vi "Close Handle.vi"(8 "error in (no error)":errorcluster, 11 "HTTP Client Base in":refnum<class "HTTP Client Base.lvclass">) -> (0 "error out":errorcluster, 3 "HTTP Client Base out":refnum<class "HTTP Client Base.lvclass">)   [LabVIEW 2021, in "HTTP Client Base.lvclass"]
uses:
  HTTP Client Base.lvclass
  HTTP Client Base.lvclass/HTTP Client Base.ctl
  <vilib>/httpClient/ClientHandle.ctl
  <vilib>/httpClient/LabVIEWHTTPClient.lvlib
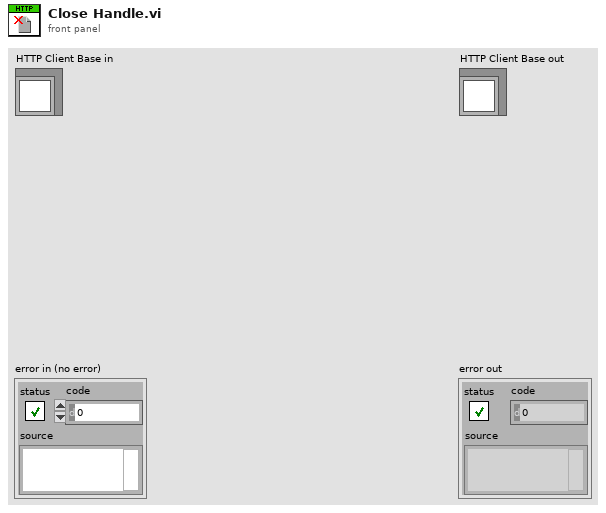
[diagram p1: front panel]
types:
  T1 = typedef "LabVIEWHTTPClient.lvlib/ClientHandle.ctl" = refnum<k1>
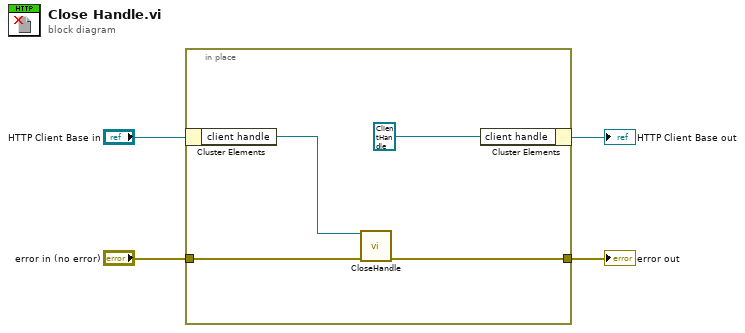
[diagram p0: block diagram]
diagram:
  n1 = in-place {
    in-place-border: "error in (no error)" -> [w8]
    in-place-border: [w7] -> w1
    n2 = in-place-cluster #1("HTTP Client Base in") -> ("client handle"=w6:T1)
    n3 = call <vilib>:"CloseHandle.vi"("client handle"=w6, "error in (no error)"=w8) -> ("error out"=w7:errorcluster)  [unwired: 13 in]
    n4 = in-place-cluster #1("client handle"=T1 refnum) -> (→"HTTP Client Base out":refnum<class "HTTP Client Base.lvclass">)
  }
  "error out" <- w1
